vi "rc_dc jack voltage.vi"(8 "error in (no error)":errorcluster) -> (0 "error out":errorcluster, 3 "function return":sgl)   [LabVIEW 2014, in "libroboticscape.lvlib"]
doc: "float get_dc_jack_voltage();"
uses:
  libroboticscape.lvlib
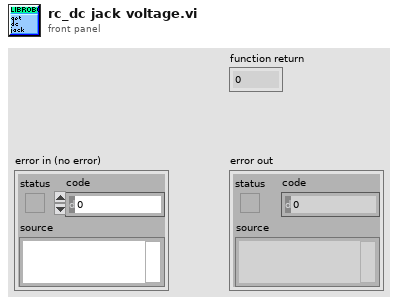
[diagram p1: front panel]
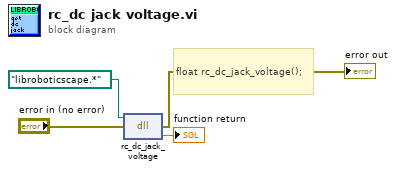
[diagram p0: block diagram]
diagram:
  # "float rc_dc_jack_voltage();"
  n1 = dll-call lib="C:/Users/ktalke/Documents/Robotics-Cape-Master-Jessie/Libroboticscape-Master-Jessie/libroboticscape.so" fn="rc_dc_jack_voltage"(path in=path "libroboticscape.*", error in="error in (no error)") -> (error out=→"error out":errorcluster, "return type"=→"function return":sgl)  [unwired: 1 in, 1 out]
